vi "OP500ZP_CLUSTER_ISO.vi"(5 "Tableau 3":string[][](array[string]), 10 "Numérique en entrée":i32, 11 "MESURES ISO":cluster{string, string}) -> (1 "Chaîne":string, 2 "Tableau 2":string[][](array[string]), 3 "Numérique en sortie":i32, 4 "Tableau":bool[](array[boolean]))   [LabVIEW 2020]
uses:
  VG/PackType.vi
  OP500ZP_VGConf.vi
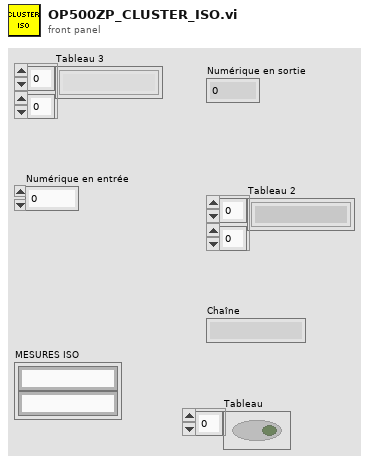
[diagram p1: front panel]
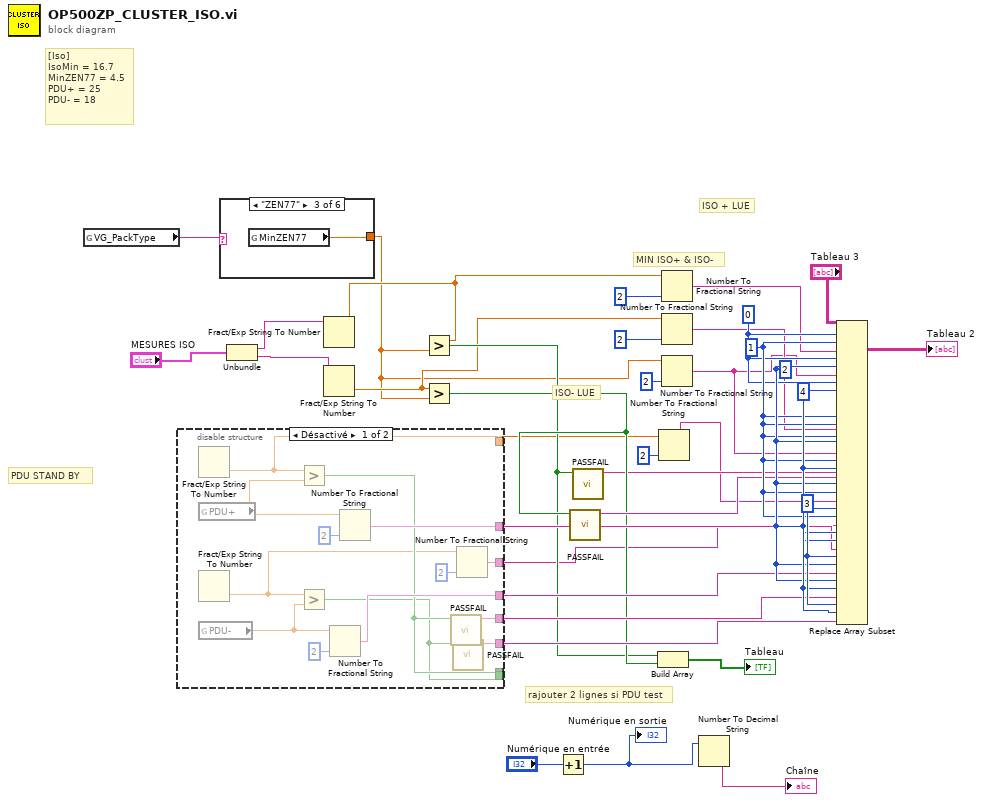
[diagram p0: block diagram]
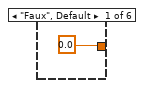
[diagram p3: hidden frame]
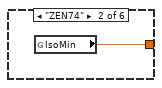
[diagram p4: hidden frame]
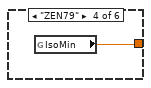
[diagram p5: hidden frame]
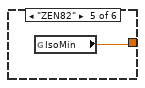
[diagram p6: hidden frame]
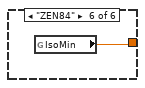
[diagram p7: hidden frame]
diagram:
  w36 = 3 ("indice désactivé (ligne)")
  w35 = 4 ("disabled index (col)")
  w34 = 2 ("disabled index (col)")
  w29 = 1 ("disabled index (col)")
  w23 = 0 ("index (row)")
  # "rajouter 2 lignes si PDU test"
  # "PDU STAND BY"
  # "[Iso]\nIsoMin = 16.7\nMinZEN77 = 4.5\nPDU+ = 25\nPDU- = 18"
  # "ISO- LUE"
  # "ISO + LUE"
  # "MIN ISO+ & ISO-"
  n1 = global read "PackType.vi" "VG_PackType"() -> (w13:string)
  n2 = disable-structure shown="Désactivé" {
    disable-tunnel: [w50 _] -> w33
    disable-tunnel: [w49 _] -> w32
    disable-tunnel: [w48 _] -> w31
    disable-tunnel: [w47 _] -> w30
    disable-tunnel: [w46 _] -> _
    disable-tunnel: [w45 _] -> _
    disable-tunnel: [w44 _] -> w7
    disable-tunnel: [w39 _] -> w2
    frame Disabled {
      n3 = Fract/Exp String To Number() -> (number=w39:dbl)  [unwired: 4 in, 1 out]
      n4 = global read "OP500ZP_VGConf.vi" "PDU+"() -> (w42:dbl)
      n5 = Fract/Exp String To Number() -> (number=w38:dbl)  [unwired: 4 in, 1 out]
      n6 = global read "OP500ZP_VGConf.vi" "PDU-"() -> (w43:dbl)
      n7 = Greater?(x=w39, y=w42) -> (0:w46:bool)
      n8 = Greater?(x=w38, y=w43) -> (0:w45:bool)
      n9 = Number To Fractional String(number=w43, precision (6)=i16 2 ("précision (6)")) -> (F-format string=w48:string)  [unwired: 2 in]
      n10 = Number To Fractional String(number=w42, precision (6)=i16 2 ("précision (6)")) -> (F-format string=w47:string)  [unwired: 2 in]
      n11 = call <userlib>:"PASSFAIL.vi"("E"=w46) -> ("S"=w49:string)  [unwired: 10 in]
      n12 = call <userlib>:"PASSFAIL.vi"("E"=w45) -> ("S"=w50:string)  [unwired: 10 in]
      n13 = Number To Fractional String(number=w38, precision (6)=i16 2 ("précision (6)")) -> (F-format string=w44:string)  [unwired: 2 in]
    }
    frame Enabled {
    }
  }
  n14 = case shown="\"ZEN77\"" w13 {
    tunnel: [0.0 ("IsoMin") w52 w53 w54 w55 w56] -> w4
    frame "Faux", Default {
    }
    frame "ZEN74" {
      n15 = global read "OP500ZP_VGConf.vi" "IsoMin"() -> (w52:dbl)
    }
    frame "ZEN77" {
      n16 = global read "OP500ZP_VGConf.vi" "MinZEN77"() -> (w53:dbl)
    }
    frame "ZEN79" {
      n17 = global read "OP500ZP_VGConf.vi" "IsoMin"() -> (w54:dbl)
    }
    frame "ZEN82" {
      n18 = global read "OP500ZP_VGConf.vi" "IsoMin"() -> (w55:dbl)
    }
    frame "ZEN84" {
      n19 = global read "OP500ZP_VGConf.vi" "IsoMin"() -> (w56:dbl)
    }
  }
  n20 = Unbundle("MESURES ISO") -> (w15:string, w14:string)
  n21 = Fract/Exp String To Number(string=w15) -> (number=w12:dbl)  [unwired: 3 in, 1 out]
  n22 = Fract/Exp String To Number(string=w14) -> (number=w10:dbl)  [unwired: 3 in, 1 out]
  n23 = Greater?(x=w12, y=w4) -> (0:w24:bool)
  n24 = Greater?(x=w10, y=w4) -> (0:w26:bool)
  n25 = Increment(x="Numérique en entrée") -> (x+1=w27:i32)
  "Numérique en sortie" <- w27
  n26 = call <userlib>:"PASSFAIL.vi"("E"=w26) -> ("S"=w28:string)  [unwired: 10 in]
  n27 = call <userlib>:"PASSFAIL.vi"("E"=w24) -> ("S"=w25:string)  [unwired: 10 in]
  n28 = Build Array(w24, w26) -> (→"Tableau":bool[])
  n29 = Number To Fractional String(number=w2, precision (6)=i16 2 ("précision (6)")) -> (F-format string=w8:string)  [unwired: 2 in]
  n30 = Number To Fractional String(number=w12, precision (6)=i16 2) -> (F-format string=w6:string)  [unwired: 2 in]
  n31 = Number To Fractional String(number=w10, precision (6)=i16 2) -> (F-format string=w9:string)  [unwired: 2 in]
  n32 = Number To Fractional String(number=w4, precision (6)=i16 2 ("précision (6)")) -> (F-format string=w3:string)  [unwired: 2 in]
  n33 = Number To Decimal String(number=w27) -> (decimal integer string=→"Chaîne":string)  [unwired: 1 in]
  n34 = Replace Array Subset(array="Tableau 3", new element #1=w6, index (row) #1=w23, index (col) #1=w29, new element #2=w3, index (row) #2=w23, index (col) #2=w34, new element #3=w25, index (row) #3=w23, index (col) #3=w35, new element #4=w9, index (row) #4=w29, index (col) #4=w29, new element #5=w3, index (row) #5=w29, index (col) #5=w34, new element #6=w28, index (row) #6=w29, index (col) #6=w35, new element #7=w8, index (row) #7=w34, index (col) #7=w29, new element #8=w7, index (row) #8=w36, index (col) #8=w29, new element #9=w30, index (row) #9=w34, index (col) #9=w34, new element #10=w31, index (row) #10=w36, index (col) #10=w34, new element #11=w32, index (row) #11=w34, index (col) #11=w35, new element #12=w33, index (row) #12=w36, index (col) #12=w35) -> (→"Tableau 2":string[][])
